vi "Format.vi"(8 "Error in (no error)":errorcluster, 10 "Log in":T1 {"Priority" items=["EMERGENCY", "ALERT", "CRITICAL", "ERROR", "WARNING", "NOTICE", "INFO", "DEBUG"]}, 11 "LogFormatterXml in":refnum<class "LogFormatterXml.lvclass">) -> (0 "Error out":errorcluster, 2 "Log formatted":string, 3 "LogFormatterXml out":refnum<class "LogFormatterXml.lvclass">)   [LabVIEW 2011, in "LogFormatterXml.lvclass"]
uses:
  LogFormatterXml.lvclass
  Log/LogCluster.ctl
  Log/PrioritiesRing.ctl
  LogFormatterXml.lvclass/LogFormatterXml.ctl
  LogFormatterSimple/LogFormatterSimple.lvclass
  Log/Log.lvclass
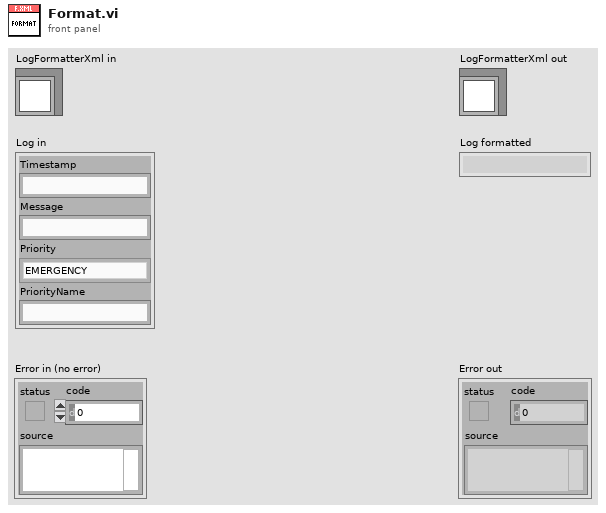
[diagram p1: front panel]
types:
  T1 = typedef "Log.lvclass/LogCluster.ctl" = cluster{"Timestamp":string, "Message":string, "Priority":T2, "PriorityName":string}
  T2 = typedef "Log.lvclass/PrioritiesRing.ctl" = u32
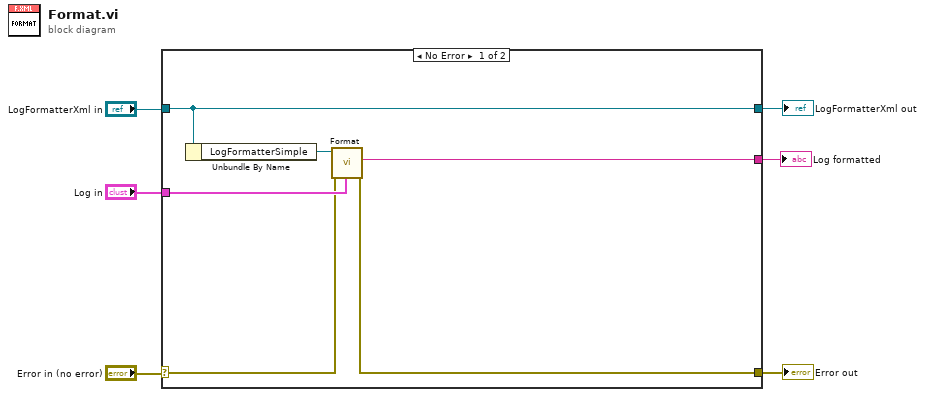
[diagram p0: block diagram]
diagram:
  n1 = case shown="No Error" "Error in (no error)" {
    selector: "Error in (no error)" -> [w9 w14]
    tunnel: [w8 w14] -> w5
    tunnel: [w12 w13] -> w3
    tunnel: "LogFormatterXml in" -> [w12 w13]
    tunnel: "Log in" -> [w10 _]
    tunnel: [w7 _] -> w1
    frame No Error {
      n2 = Unbundle By Name(w12) -> ("LogFormatterSimple"=w11:refnum<class "LogFormatterSimple.lvclass">)
      n3 = call-dynamic "Format.vi"("Error in (no error)"=w9, "Log in"=w10, "LogFormatterSimple in"=w11) -> ("Error out"=w8:errorcluster, "Log formatted"=w7:string)  [unwired: 6 in, 1 out]
    }
    frame Error {
    }
  }
  "Error out" <- w5
  "LogFormatterXml out" <- w3
  "Log formatted" <- w1
